vi "Read Time Info.vi"(0 "Request Data in":refnum<class "Timed Data.lvclass">, 11 "error in (no error)":errorcluster) -> (4 "Request Data out":refnum<class "Timed Data.lvclass">, 6 "Start TIme":timestamp, 8 "Duration(s)":dbl, 10 "Data ID":u32, 15 "error out":errorcluster)   [LabVIEW 2020, in "Publisher.lvlib" / "Timed Data.lvclass"]
doc: "Read Start Time, Duration and DataID from the Timed Data."
uses:
  Timed Data.lvclass
  Timed Data.lvclass/Timed Data.ctl
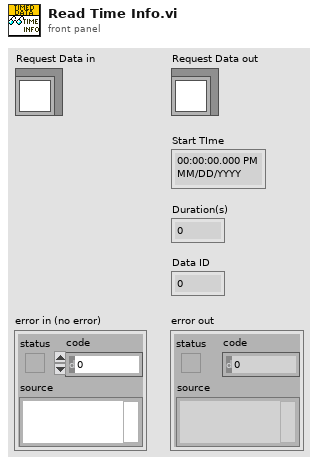
[diagram p1: front panel]
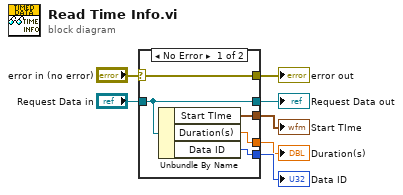
[diagram p0: block diagram]
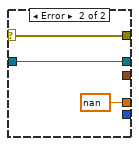
[diagram p2: hidden frame]
diagram:
  n1 = case shown="No Error" "error in (no error)" {
    selector: "error in (no error)" -> [w12 w14]
    tunnel: [w12 w14] -> w6
    tunnel: [w11 w15] -> w4
    tunnel: "Request Data in" -> [w11 w15]
    tunnel: [w10 _] -> w3
    tunnel: [w9 _] -> w2
    tunnel: [w8 nan ("Duration(s)")] -> w1
    frame No Error {
      n2 = Unbundle By Name(w11) -> ("Start TIme"=w9:timestamp, "Duration(s)"=w8:dbl, "Data ID"=w10:u32)
    }
    frame Error {
    }
  }
  "error out" <- w6
  "Request Data out" <- w4
  "Data ID" <- w3
  "Start TIme" <- w2
  "Duration(s)" <- w1
